vi "Raw Values.vi"(8 "error in (no error)":errorcluster, 11 "Message Queues":T1) -> ()   [LabVIEW 2023, in "Weather Monitor Views.lvlib"]
doc: "Calls the Weather Monitor web service with different content-types and displays the raw data that is returned."
uses:
  Weather Monitor Views.lvlib
  support/Message Queue/All Message Queues.ctl
  support/Message Queue/Message Cluster.ctl
  Request/Response Data.ctl
  support/Message Queue/Weather Message Queue.lvlib
  Weather Request Loop.lvlib
  support/User Event - Stop/Weather User Event - Stop.lvlib
panel:
  out "Last Content Type":string
  in  "Close button":bool
  out "Weather data":string
  out "Last Response Code":u16
  in  "Data Type":string(combo)="application/json" caption="Data Content Type"
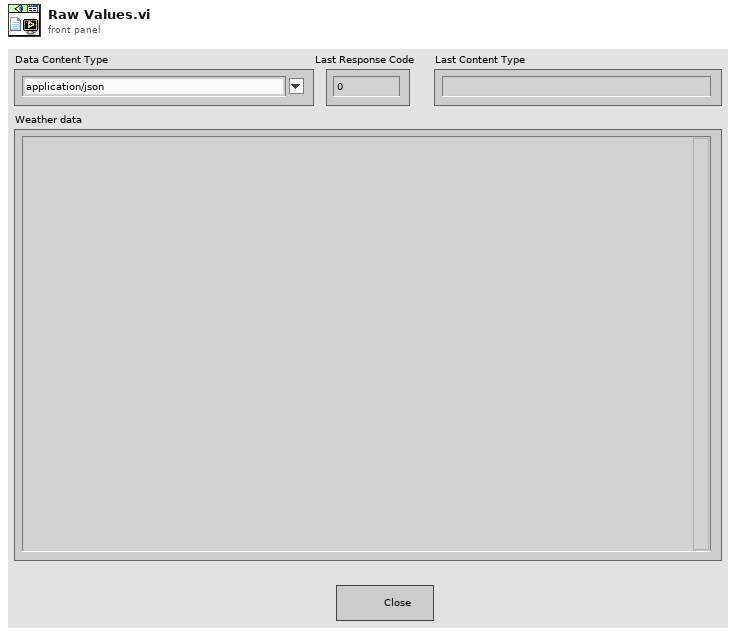
[diagram p1: front panel]
types:
  T1 = typedef "Weather Message Queue.lvlib/All Message Queues.ctl" = cluster{"View":refnum<queue>, "Request":refnum<queue>, "Wait":refnum<queue>}
  T2 = typedef "Weather Request Loop.lvlib/Response Data.ctl" = cluster{"Response Code":u16, "Body":string, "Headers":variant, "error":errorcluster}
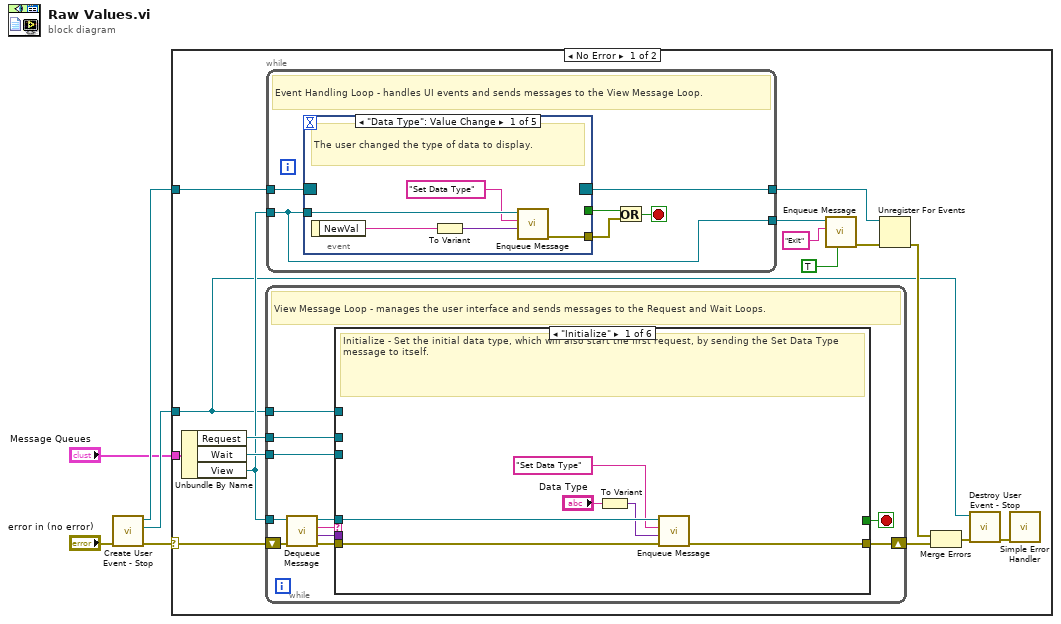
[diagram p0: block diagram]
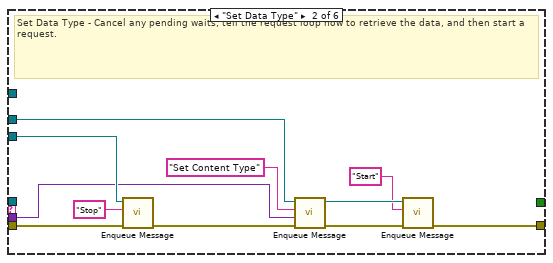
[diagram p2: hidden frame]
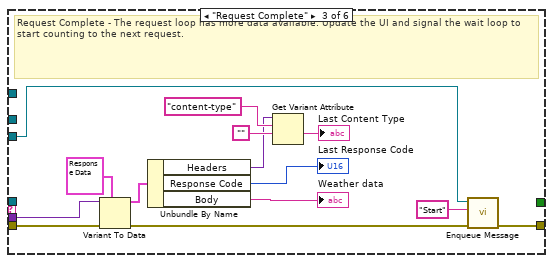
[diagram p3: hidden frame]
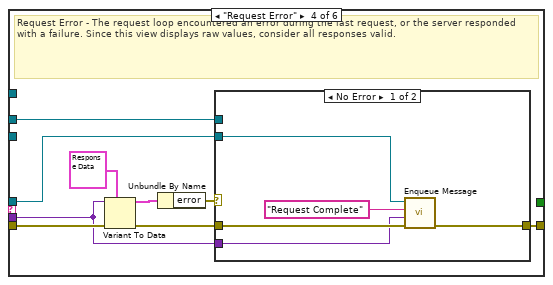
[diagram p4: hidden frame]
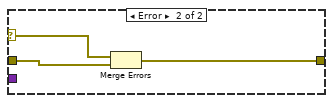
[diagram p5: hidden frame]
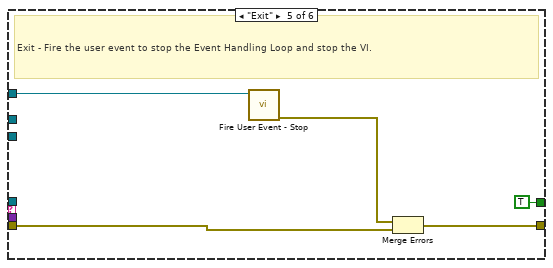
[diagram p6: hidden frame]
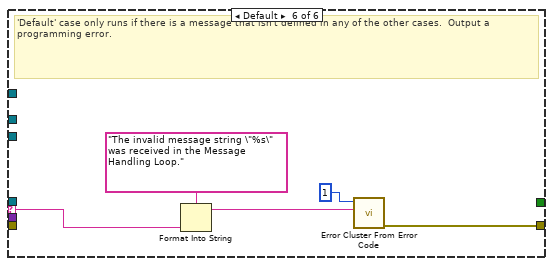
[diagram p7: hidden frame]
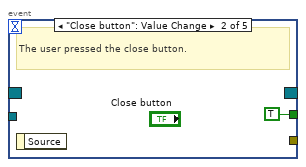
[diagram p8: hidden frame]
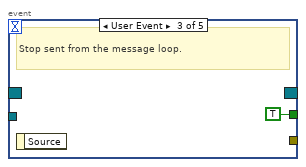
[diagram p9: hidden frame]
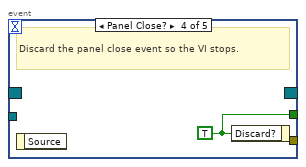
[diagram p10: hidden frame]
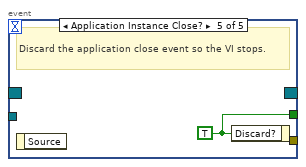
[diagram p11: hidden frame]
diagram:
  n1 = call "Create User Event - Stop.vi"("error in (no error)"="error in (no error)") -> ("error out"=w4:errorcluster, "User Event - Stop"=w2:refnum<user-event>, "Stop Event Registration Refnum"=w3:refnum<event-registration>)  [unwired: 8 in]
  n2 = case shown="No Error" w4 {
    selector: w4 -> [w16 _]
    tunnel: "Message Queues" -> [w21 _]
    tunnel: w3 -> [w15 _]
    tunnel: w2 -> [w10 _]
    frame No Error {
      n3 = Unbundle By Name(w21) -> ("Request"=w20:refnum<queue>, "Wait"=w19:refnum<queue>, "View"=w18:refnum<queue>)
      n4 = while {
        tunnel: w20 -> [w24]
        tunnel: w19 -> [w25]
        tunnel: w18 -> [w32]
        shift-right: [w26] -> w17
        shift-left: w16 -> [w31]
        tunnel: w10 -> [w22]
        stop <- w23 stop-if-true
        # "View Message Loop - manages the user interface and sends messages to the Request and Wait Loops."
        n5 = call "Dequeue Message.vi"("error in (no error)"=w31, "Message Queue"=w32) -> ("error out"=w27:errorcluster, "Message Data"=w28:variant, "Message"=w30:string, "dup Message Queue"=w29:refnum<queue>)  [unwired: 6 in]
        n6 = case shown="\"Initialize\"" w30 {
          selector: w30 -> [_ _ _ _ _ w87]
          tunnel: w29 -> [w36 _ _ w65 _ _]
          tunnel: w28 -> [_ w39 w62 w64 _ _]
          tunnel: w27 -> [w38 w49 w63 w72 w81 _]
          tunnel: [w37 w43 w58 w68 w82 w86] -> w26
          tunnel: w25 -> [_ w41 w57 _ _ _]
          tunnel: w24 -> [_ w48 _ w67 _ _]
          tunnel: [_ _ _ _ TRUE _] -> w23
          tunnel: w22 -> [_ _ _ _ w84 _]
          frame "Initialize" {
            # "Initialize - Set the initial data type, which will also start the first request, by sending the Set Data Type message to itself."
            n7 = To Variant(anything="Data Type") -> (Variant=w34:variant)
            n8 = call "Enqueue Message.vi"("error in (no error)"=w38, "Message Data"=w34, "Message"="Set Data Type", "Message Queue"=w36) -> ("error out"=w37:errorcluster)  [unwired: 6 in, 1 out]
          }
          frame "Set Data Type" {
            # "Set Data Type - Cancel any pending waits, tell the request loop how to retrieve the data, and then start a request."
            n9 = call "Enqueue Message.vi"("error in (no error)"=w49, "Message"="Stop", "Message Queue"=w41) -> ("error out"=w42:errorcluster)  [unwired: 7 in, 1 out]
            n10 = call "Enqueue Message.vi"("error in (no error)"=w42, "Message Data"=w39, "Message"="Set Content Type", "Message Queue"=w48) -> ("error out"=w45:errorcluster, "dup Message Queue"=w46:refnum<queue>)  [unwired: 6 in]
            n11 = call "Enqueue Message.vi"("error in (no error)"=w45, "Message"="Start", "Message Queue"=w46) -> ("error out"=w43:errorcluster)  [unwired: 7 in, 1 out]
          }
          frame "Request Complete" {
            # "Request Complete - The request loop has more data available. Update the UI and signal the wait loop to start counting to the next request."
            n12 = Variant To Data(error in=w63, type=T2 {"Response Code"=0, "Body"="", "Headers"=variant, "error"={"status"=FALSE, "code"=0, "source"=""}} ("Response Data"), Variant=w62) -> (data=w60:T2, error out=w59:errorcluster)
            n13 = Unbundle By Name(w60) -> ("Headers"=w51:variant, "Response Code"=→"Last Response Code":u16, "Body"=→"Weather data":string)
            n14 = Get Variant Attribute(Variant=w51, name="content-type", default value (empty Variant)="") -> (value=→"Last Content Type":string)  [unwired: 1 in, 3 out]
            n15 = call "Enqueue Message.vi"("error in (no error)"=w59, "Message"="Start", "Message Queue"=w57) -> ("error out"=w58:errorcluster)  [unwired: 7 in, 1 out]
          }
          frame "Request Error" {
            # "Request Error - The request loop encountered an error during the last request, or the server responded with a failure. Since this view displays raw values, consider all responses valid."
            n16 = Variant To Data(error in=w72, type=T2 {"Response Code"=0, "Body"="", "Headers"=variant, "error"={"status"=FALSE, "code"=0, "source"=""}} ("Response Data"), Variant=w64) -> (data=w66:T2, error out=w70:errorcluster)
            n17 = Unbundle By Name(w66) -> ("error"=w69:errorcluster)
            n18 = case shown="No Error" w69 {
              selector: w69 -> [_ w80]
              tunnel: w70 -> [w77 w78]
              tunnel: [w76 w79] -> w68
              tunnel: w67 -> [_ _]
              tunnel: w65 -> [w75 _]
              tunnel: w64 -> [w74 _]
              frame No Error {
                n19 = call "Enqueue Message.vi"("error in (no error)"=w77, "Message Data"=w74, "Message"="Request Complete", "Message Queue"=w75) -> ("error out"=w76:errorcluster)  [unwired: 6 in, 1 out]
              }
              frame Error {
                n20 = Merge Errors(w80, w78) -> (w79:errorcluster)
              }
            }
          }
          frame "Exit" {
            # "Exit - Fire the user event to stop the Event Handling Loop and stop the VI."
            n21 = call "Fire User Event - Stop.vi"("User Event - Stop"=w84) -> ("error out"=w83:errorcluster)  [unwired: 10 in]
            n22 = Merge Errors(w83, w81) -> (w82:errorcluster)
          }
          frame Default {
            # "'Default' case only runs if there is a message that isn't defined in any of the other cases.  Output a programming error."
            n23 = Format Into String(format string="The invalid message string \"%s\" was received in the Message Handling Loop." ("Unknown Message Error Text"), w87) -> (resulting string=w88:string)  [unwired: 2 in, 1 out]
            n24 = call <vilib>:"Error Cluster From Error Code.vi"("error message (\"\")"=w88, "error code (0)"=1) -> ("error out"=w86:errorcluster)  [unwired: 7 in]
          }
        }
      }
      n25 = while {
        tunnel: w18 -> [w94]
        tunnel: w15 -> [w96]
        tunnel: [w95] -> w13
        tunnel: [w94] -> w6
        stop <- w92 stop-if-true
        # "Event Handling Loop - handles UI events and sends messages to the View Message Loop."
        n26 = event shown="[0] \"Data Type\": Value Change" {
          selector: w96 -> [_ _ _ _ _]
          dyn-events: [_ _ _ _ _] -> w95
          timeout: _ -> [_ _ _ _ _]
          tunnel: w94 -> [w101 _ _ _ _]
          tunnel: [w97 _ _ _ _] -> w91
          tunnel: [_ TRUE TRUE w104 w105] -> w93
          event "Data Type": Value Change {
            # "The user changed the type of data to display."
            n27 = event-data() -> ("NewVal"=w99:string)  [unwired: 1 in]
            n28 = To Variant(anything=w99) -> (Variant=w98:variant)
            n29 = call "Enqueue Message.vi"("Message Data"=w98, "Message"="Set Data Type", "Message Queue"=w101) -> ("error out"=w97:errorcluster)  [unwired: 7 in, 1 out]
          }
          event "Close button": Value Change {
            # "The user pressed the close button."
            n30 = event-data() -> ()  [unwired: 1 in, 1 out]
          }
          event User Event {
            # "Stop sent from the message loop."
            n31 = event-data() -> ()  [unwired: 1 in, 1 out]
          }
          event Panel Close? {
            w104 = TRUE ("Discard?")
            # "Discard the panel close event so the VI stops."
            n32 = event-data() -> ()  [unwired: 1 in, 1 out]
            n33 = event-data("Discard?"=w104) -> ()  [unwired: 1 in, 1 out]
          }
          event Application Instance Close? {
            w105 = TRUE ("Discard?")
            # "Discard the application close event so the VI stops."
            n34 = event-data() -> ()  [unwired: 1 in, 1 out]
            n35 = event-data("Discard?"=w105) -> ()  [unwired: 1 in, 1 out]
          }
        }
        n36 = Or(x=w93, y=w91) -> (x .or. y?=w92:bool)
      }
      n37 = call "Enqueue Message.vi"("Priority Message? (F)"=TRUE, "Message"="Exit", "Message Queue"=w6) -> ("error out"=w7:errorcluster)  [unwired: 7 in, 1 out]
      n38 = Unregister For Events(event registration refnum=w13, error in=w7) -> (error out=w14:errorcluster)
      n39 = Merge Errors(w14, w17) -> (w12:errorcluster)
      n40 = call "Destroy User Event - Stop.vi"("error in (no error)"=w12, "User Event - Stop"=w10) -> ("error out"=w11:errorcluster)  [unwired: 9 in]
      n41 = call <vilib>:"Simple Error Handler.vi"("error in (no error)"=w11) -> ()  [unwired: 4 in, 5 out]
    }
    frame Error {
    }
  }
